vi "Create Virtual FolderItem.vi"(8 "error in (no error)":errorcluster, 10 "Folder Name":string, 11 "ProjectItem in":refnum<vi>) -> (0 "error out":errorcluster, 1 "Already exists?":bool, 2 "FolderItem reference out":refnum<vi>, 3 "ProjectItem out":refnum<vi>)   [LabVIEW 2019, in "gRPC Template Creation Utility.lvlib"]
uses:
  gRPC Template Creation Utility.lvlib
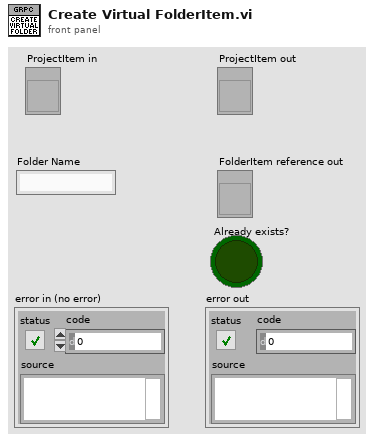
[diagram p1: front panel]
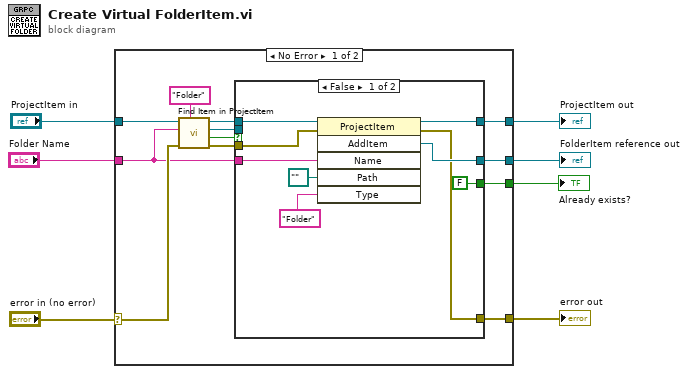
[diagram p0: block diagram]
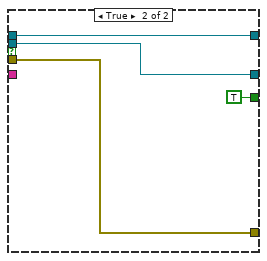
[diagram p2: hidden frame]
diagram:
  n1 = case shown="No Error" "error in (no error)" {
    selector: "error in (no error)" -> [w14 w33]
    tunnel: [w19 _] -> w7
    tunnel: [w18 w34] -> w2
    tunnel: "Folder Name" -> [w8 _]
    tunnel: "ProjectItem in" -> [w16 w34]
    tunnel: [w17 w33] -> w5
    tunnel: [w10 _] -> w1
    frame No Error {
      n2 = call "Find Item in ProjectItem.vi"("Item Type"="Folder" ("Type"), "error in (no error)"=w14, "Name"=w8, "ProjectItem in"=w16) -> ("error out"=w9:errorcluster, "Found ?"=w13:bool, "Item Refnum out"=w11:refnum<vi>, "ProjectItem out"=w12:refnum<vi>)  [unwired: 4 in]
      n3 = case shown="False" w13 {
        tunnel: [w28 w32] -> w19
        tunnel: [w27 w31] -> w18
        tunnel: [w25 w30] -> w17
        tunnel: w12 -> [w24 w31]
        tunnel: w11 -> [_ w32]
        tunnel: [FALSE TRUE] -> w10
        tunnel: w9 -> [w23 w30]
        tunnel: w8 -> [w21 _]
        frame False {
          n4 = invoke class="ProjectItem" method="AddItem"(reference=w24, error in=w23, "Name"=w21, "Path"=path "", "Type"="Folder") -> (reference out=w27:refnum<vi>, error out=w25:errorcluster, "AddItem"=w28:refnum<vi>)  [unwired: 1 in, 3 out]
        }
        frame True {
        }
      }
    }
    frame Error {
    }
  }
  "FolderItem reference out" <- w7
  "error out" <- w5
  "ProjectItem out" <- w2
  "Already exists?" <- w1
